vi "Align PID Tuner.vi"(2 "Current Position":cluster{"X":dbl, "Y":dbl, "Theta":dbl}, 3 "Debug Input":T2, 4 "Final Position":cluster{"X":dbl, "Y":dbl, "Theta":dbl}) -> (0 "Graph Data":cluster{"Error":dbl, "Exppected":dbl}, 1 "Sine Corrected Positions":cluster{"X":dbl, "Y":dbl, "Theta":dbl})   [LabVIEW 2025]
uses:
  Implementation/Tune Auto Pickup PID.ctl
  <vilib>/ptbypt/NI_PtbyPt.lvlib
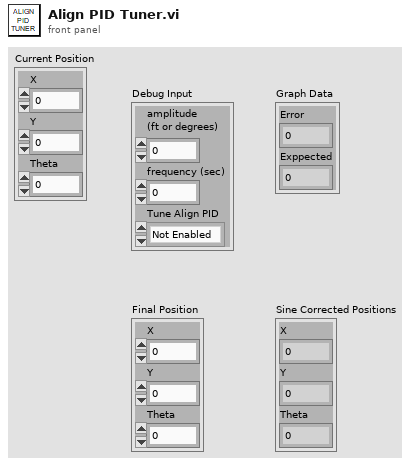
[diagram p1: front panel]
types:
  T1 = typedef "Tune Auto Pickup PID.ctl" = enum16{"Not Enabled", "X Axis", "Y Axis", "Theta"}
  T2 = cluster{"amplitude \n(ft or degrees)":dbl, "frequency (sec)":dbl, "Tune Align PID":T1}
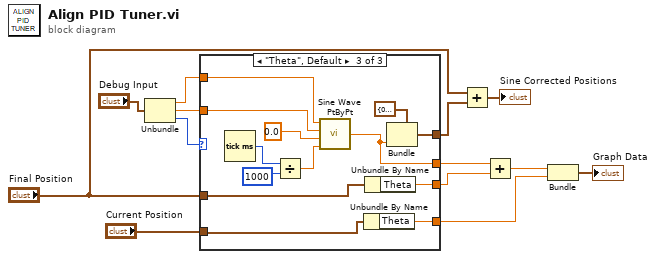
[diagram p0: block diagram]
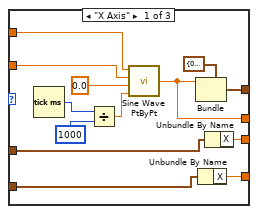
[diagram p2: hidden frame]
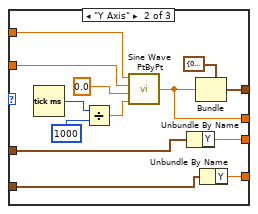
[diagram p3: hidden frame]
diagram:
  n1 = Unbundle("Debug Input") -> ("amplitude \n(ft or degrees)"=w13:dbl, "frequency (sec)"=w12:dbl, "Tune Align PID"=w11:T1)
  n2 = case shown="\"Theta\", Default" w11 {
    tunnel: [w25 w38 w51] -> w3
    tunnel: w13 -> [w23 w36 w49]
    tunnel: w12 -> [w22 w35 w48]
    tunnel: [w21 w34 w47] -> w9
    tunnel: [w20 w33 w46] -> w7
    tunnel: "Final Position" -> [w16 w29 w42]
    tunnel: [w14 w28 w41] -> w5
    tunnel: "Current Position" -> [w15 w27 w40]
    frame "X Axis" {
      n3 = Tick Count (ms)() -> (millisecond timer value=w18:u32)
      n4 = Divide(x=w18, y=u32 1000) -> (x/y=w17:dbl)
      n5 = call <vilib>:"Sine Wave PtByPt.vi"("time"=w17, "phase"=0.0, "frequency"=w22, "amplitude"=w23) -> ("sine wave"=w21:dbl)
      n6 = Bundle(cluster=cluster{"X":dbl, "Y":dbl, "Theta":dbl} {"X"=0.0, "Y"=0.0, "Theta"=0.0}, "X"=w21) -> (w25:cluster{"X":dbl, "Y":dbl, "Theta":dbl})  [unwired: 2 in]
      n7 = Unbundle By Name(w15) -> ("X"=w14:dbl)
      n8 = Unbundle By Name(w16) -> ("X"=w20:dbl)
    }
    frame "Y Axis" {
      n9 = Tick Count (ms)() -> (millisecond timer value=w30:u32)
      n10 = Divide(x=w30, y=u32 1000) -> (x/y=w31:dbl)
      n11 = call <vilib>:"Sine Wave PtByPt.vi"("time"=w31, "phase"=0.0, "frequency"=w35, "amplitude"=w36) -> ("sine wave"=w34:dbl)
      n12 = Unbundle By Name(w29) -> ("Y"=w33:dbl)
      n13 = Bundle(cluster=cluster{"X":dbl, "Y":dbl, "Theta":dbl} {"X"=0.0, "Y"=0.0, "Theta"=0.0}, "Y"=w34) -> (w38:cluster{"X":dbl, "Y":dbl, "Theta":dbl})  [unwired: 2 in]
      n14 = Unbundle By Name(w27) -> ("Y"=w28:dbl)
    }
    frame "Theta", Default {
      n15 = Tick Count (ms)() -> (millisecond timer value=w44:u32)
      n16 = Divide(x=w44, y=u32 1000) -> (x/y=w45:dbl)
      n17 = call <vilib>:"Sine Wave PtByPt.vi"("time"=w45, "phase"=0.0, "frequency"=w48, "amplitude"=w49) -> ("sine wave"=w47:dbl)
      n18 = Unbundle By Name(w40) -> ("Theta"=w41:dbl)
      n19 = Unbundle By Name(w42) -> ("Theta"=w46:dbl)
      n20 = Bundle(cluster=cluster{"X":dbl, "Y":dbl, "Theta":dbl} {"X"=0.0, "Y"=0.0, "Theta"=0.0}, "Theta"=w47) -> (w51:cluster{"X":dbl, "Y":dbl, "Theta":dbl})  [unwired: 2 in]
    }
  }
  n21 = Add(x="Final Position", y=w3) -> (x+y=→"Sine Corrected Positions":cluster{"X":dbl, "Y":dbl, "Theta":dbl})
  n22 = Add(x=w9, y=w7) -> (x+y=w8:dbl)
  n23 = Bundle(w8, "Theta"=w5) -> (→"Graph Data":cluster{dbl, "Theta":dbl})  [unwired: 1 in]
